vi "Main.vi"() -> ()   [LabVIEW 2011]
panel:
  out "Output":string
  # "This is the Main vi\nIt now does something"
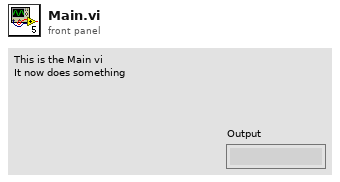
[diagram p1: front panel]
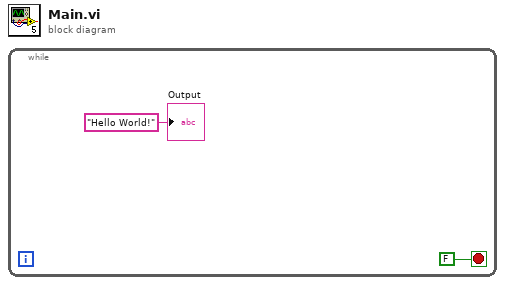
[diagram p0: block diagram]
diagram:
  n1 = while {
    stop <- FALSE stop-if-true
    "Output" <- "Hello World!" ("Output")
  }
